vi "Graph Sine Array (Completed - 2D Array).vi"() -> ()   [LabVIEW 2018]
doc: "This VI generates a sine wave and a cosine wave and plots them on a waveform graph."
uses:
  <vilib>/Utility/file.llb/Write Delimited Spreadsheet (DBL).vi
panel:
  out "Waveform Array":dbl[](array[numeric]) format="%.2f"
  out "Waveform Graph":dbl[][](graph)
  # "*Digital Indicator Array*"
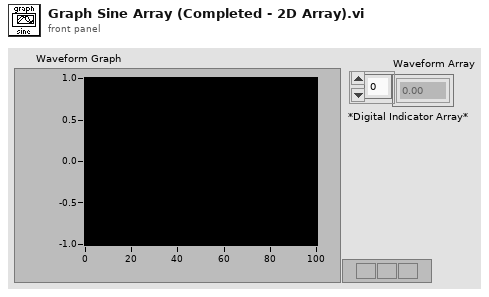
[diagram p1: front panel]
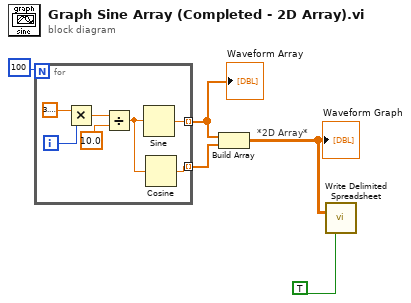
[diagram p0: block diagram]
diagram:
  # "*2D Array*"
  n1 = for {
    N: 100 -> [_]
    tunnel: [w8] -> w3 mode=indexing
    tunnel: [w6] -> w4 mode=indexing
    i -> [w11]
    n2 = Multiply(x=3.141592653589793, y=w11) -> (x*y=w10:dbl)
    n3 = Divide(x=w10, y=10.0) -> (x/y=w7:dbl)
    n4 = Sine(x=w7) -> (sin(x)=w8:dbl)
    n5 = Cosine(x=w7) -> (cos(x)=w6:dbl)
  }
  "Waveform Array" <- w3
  n6 = Build Array "Build Array"(w3, w4) -> (w2:dbl[][])
  "Waveform Graph" <- w2
  n7 = call-poly <vilib>:"Write Delimited Spreadsheet.vi"("2D data"=w2, "transpose? (no:F)"=TRUE) -> ()  [unwired: 12 in, 2 out]
